vi "Get Tool Config.vi"(8 "error in (no error)":errorcluster, 10 "dummy":bool) -> (0 "error out":errorcluster, 1 "timed out?":bool, 2 "Reply Payload":T1={"Version String"="", "Tool Config"={"Tool Type"=0, "Tool SN"=0, "Tool Block"={"Encoder Size"=0, "Encoder Scale"=0, "Encoder Offset"=0, "MaxEncoder"=0, "MinEncoder"=0, "Start Delay"=0.0, "Tool Face Ref"=0.0}, "Motor Block"={"MinMotor Speed"=0, "MaxMotor Speed"=0, "Homing Speed"=90, "Jog Speed"=90, "Inspect Speed"=90, "VBlk Speed"=90, "CleaningPos"=0, "Safe Zone"=0, "Has Motor"=FALSE, "Use Home Index"=FALSE}, "Verification Block"={"Angle"=90.0, "FlankLength1"=0.0, "FlankLength2"=0.0, "Location"=0.0, "Serial Number"=0}, "Probe Block"={"nProbes"=0, "Probe Param Array"=[]}}})   [LabVIEW 2015, in "Tool Module.lvlib"]
doc: "Gets the Tool Configuration Cluster. (This copy is from the last time the app connected to the tool.)\n_____\nCreated using Delacor QMH Event Scripter 3.1.0.29."
uses:
  Tool Module.lvlib
  Get Tool Config (Reply Payload)--cluster.ctl
  Tool Config/_Configuration Cluster_v3--typedef.ctl
  Tool Config/_Tool Block Cluster_v3--typedef.ctl
  Tool Config/_Motor Block Cluster_v2--typedef.ctl
  Tool Config/_Verification Blk Cluster--typedef.ctl
  Tool Config/_ProbeConfigParams Cluster--typedef.ctl
  Tool Config/_Sensor Block Cluster--typedef.ctl
  Tool Config/_SensorConfigParams Cluster--typedef.ctl
  Get Tool Config Argument--cluster.ctl
  Tool Config/Tool Cfg.lvlib
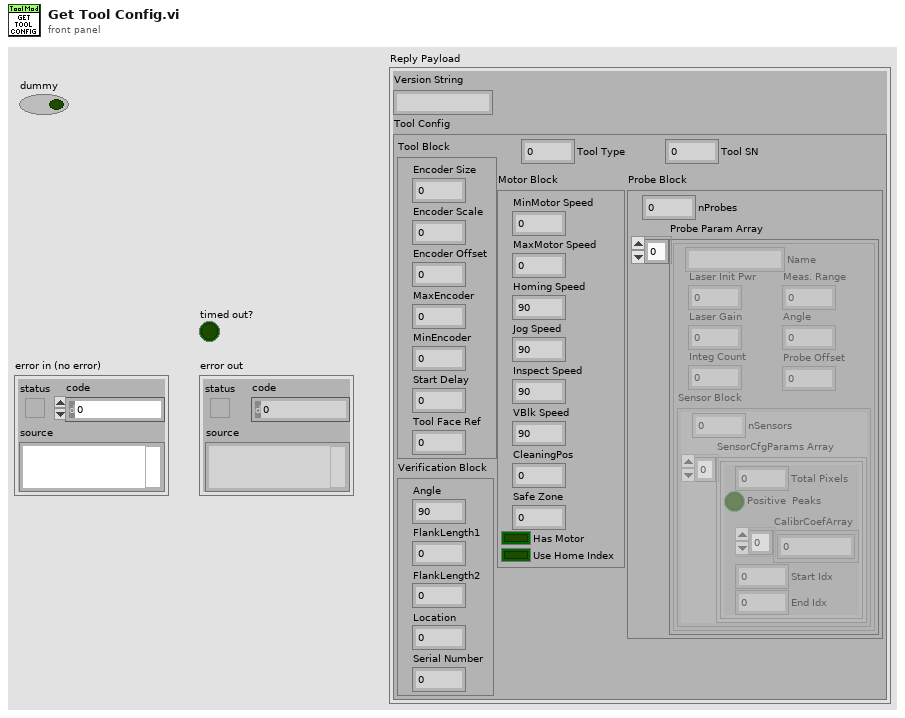
[diagram p1: front panel]
types:
  T1 = typedef "Tool Module.lvlib/Get Tool Config (Reply Payload)--cluster.ctl" = cluster{"Version String":string, "Tool Config":T2}
  T2 = typedef "Tool Cfg.lvlib/_Configuration Cluster_v3--typedef.ctl" = cluster{"Tool Type":u16, "Tool SN":u16, "Tool Block":T3, "Motor Block":T4, "Verification Block":T5, "Probe Block":cluster{"nProbes":u16, "Probe Param Array":T6[]}}
  T3 = typedef "Tool Cfg.lvlib/_Tool Block Cluster_v3--typedef.ctl" = cluster{"Encoder Size":u16, "Encoder Scale":u32, "Encoder Offset":i32, "MaxEncoder":i32, "MinEncoder":i32, "Start Delay":sgl, "Tool Face Ref":sgl}
  T4 = typedef "Tool Cfg.lvlib/_Motor Block Cluster_v2--typedef.ctl" = cluster{"MinMotor Speed":u16, "MaxMotor Speed":u16, "Homing Speed":u16, "Jog Speed":u16, "Inspect Speed":u16, "VBlk Speed":u16, "CleaningPos":i32, "Safe Zone":i32, "Has Motor":bool, "Use Home Index":bool}
  T5 = typedef "Tool Cfg.lvlib/_Verification Blk Cluster--typedef.ctl" = cluster{"Angle":sgl, "FlankLength1":sgl, "FlankLength2":sgl, "Location":sgl, "Serial Number":u16}
  T6 = typedef "Tool Cfg.lvlib/_ProbeConfigParams Cluster--typedef.ctl" = cluster{"Name":string, "Laser Init Pwr":u16, "Laser Gain":u8, "Integ Count":u16, "Meas. Range":sgl, "Angle":sgl, "Probe Offset":sgl, "Sensor Block":T7}
  T7 = typedef "Tool Cfg.lvlib/_Sensor Block Cluster--typedef.ctl" = cluster{"nSensors":u16, "SensorCfgParams Array":T8[]}
  T8 = typedef "Tool Cfg.lvlib/_SensorConfigParams Cluster--typedef.ctl" = cluster{"Total Pixels":u16, "Positive  Peaks":bool, "CalibrCoefArray":dbl[], "Start Idx":u16, "End Idx":u16}
  T9 = typedef "Tool Module.lvlib/Get Tool Config Argument--cluster.ctl" = cluster{"dummy":bool, "Wait Notifier":refnum<notifier>}
  T10 = typedef "Tool Module.lvlib/Request Events--cluster.ctl" = cluster{"Stop Module":refnum<user-event>, "Show Panel":refnum<user-event>, "Hide Panel":refnum<user-event>, "Get Module Execution Status":refnum<user-event>, "Show Diagram":refnum<user-event>, "Set OpCfg":refnum<user-event>, "Get Op Cfg":refnum<user-event>, "Test Trig 2":refnum<user-event>, "GOTO":refnum<user-event>, "Start Inspect":refnum<user-event>, "CONNECT":refnum<user-event>, "Get All Inspect Data":refnum<user-event>, "Get Inspection Limits":refnum<user-event>, "Set Inspection Limits":refnum<user-event>, "Update Status":refnum<user-event>, "Get Data Format Params":refnum<user-event>, "Start Data Monitor":refnum<user-event>, "Get FPGA Setup Params":refnum<user-event>, "Set FPGA Setup Params":refnum<user-event>, "Set Tool Config":refnum<user-event>, "Get Tool Config":refnum<user-event>, "Set Integration Count":refnum<user-event>, "Set Laser Params":refnum<user-event>, "Get Mtrl Ctrl Reg":refnum<user-event>, "Commit Ctrl Reg":refnum<user-event>, "Set Event Logger":refnum<user-event>, "Write to File":refnum<user-event>, "Read from File":refnum<user-event>, "Set Device Temp Thresholds":refnum<user-event>}
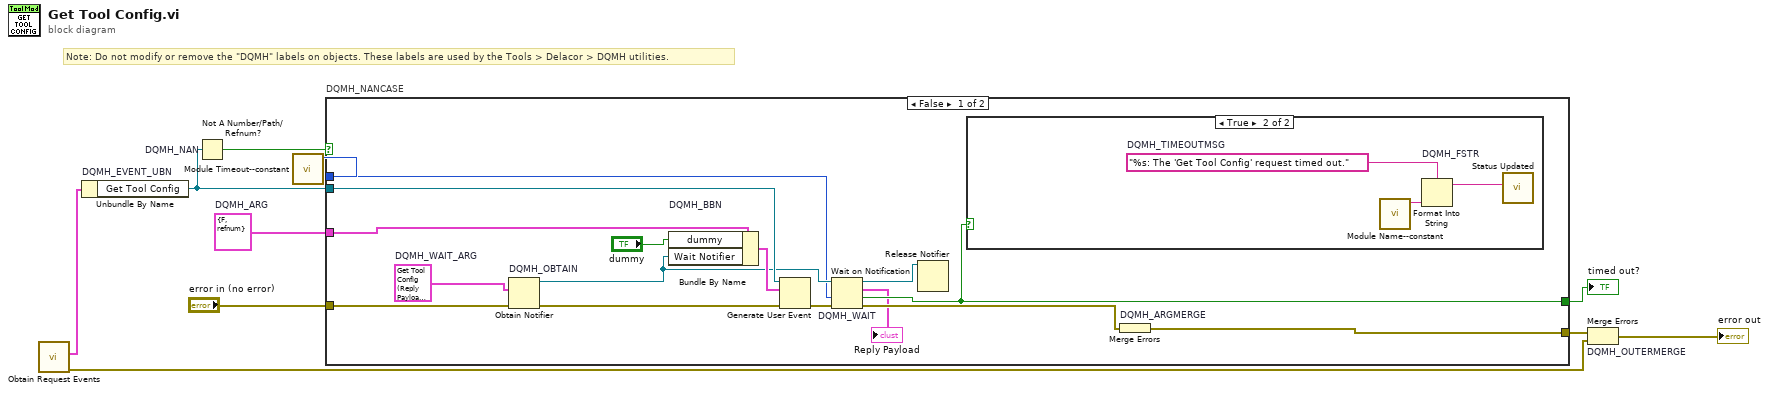
[diagram p0: block diagram]
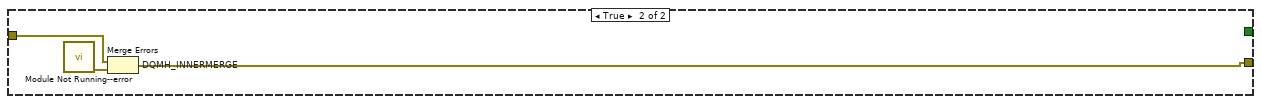
[diagram p3: hidden frame]
diagram:
  w4 = T9 {"dummy"=FALSE, "Wait Notifier"=refnum}  # DQMH_ARG
  # "Note: Do not modify or remove the \"DQMH\" labels on objects. These labels are used by the Tools > Delacor > DQMH utilities."
  n1 = call "Obtain Request Events.vi"() -> ("error out"=w2:errorcluster, "Tool Module Request Events"=w1:T10)  [unwired: 10 in]
  n2 = Unbundle By Name "DQMH_EVENT_UBN"(w1) -> ("Get Tool Config"=w8:refnum<user-event>)
  n3 = Not A Number/Path/Refnum? "DQMH_NAN"(number/path/refnum=w8) -> (NaN/Path/Refnum?=w7:bool)
  n4 = call "Module Timeout--constant.vi"() -> ("Module Timeout"=w3:i32)  [unwired: 11 in]
  n5 = case "DQMH_NANCASE" shown="False" w7 {
    tunnel: "error in (no error)" -> [w25 w31]
    tunnel: w8 -> [w23 _]
    tunnel: [w15 w30] -> w5
    tunnel: [w16 _] -> w6
    tunnel: w4 -> [w14 _]
    tunnel: w3 -> [w12 _]
    frame False {
      w20 = T1 {"Version String"="", "Tool Config"={"Tool Type"=0, "Tool SN"=0, "Tool Block"={"Encoder Size"=0, "Encoder Scale"=0, "Encoder Offset"=0, "MaxEncoder"=0, "MinEncoder"=0, "Start Delay"=0.0, "Tool Face Ref"=0.0}, "Motor Block"={"MinMotor Speed"=0, "MaxMotor Speed"=0, "Homing Speed"=90, "Jog Speed"=90, "Inspect Speed"=90, "VBlk Speed"=90, "CleaningPos"=0, "Safe Zone"=0, "Has Motor"=FALSE, "Use Home Index"=FALSE}, "Verification Block"={"Angle"=90.0, "FlankLength1"=0.0, "FlankLength2"=0.0, "Location"=0.0, "Serial Number"=0}, "Probe Block"={"nProbes"=0, "Probe Param Array"=[]}}}  # DQMH_WAIT_ARG
      n6 = Obtain Notifier "DQMH_OBTAIN"(notification data type=w20, error in (no error)=w25) -> (notifier out=w18:refnum<notifier>, error out=w21:errorcluster)  [unwired: 2 in, 1 out]
      n7 = Bundle By Name "DQMH_BBN"(cluster=w14, "dummy"="dummy", "Wait Notifier"=w18) -> (w22:T9)
      n8 = Generate User Event(user event=w23, event data cluster=w22, error in=w21) -> (error out=w24:errorcluster)  [unwired: 1 in, 1 out]
      n9 = Wait on Notification "DQMH_WAIT"(notifier=w18, timeout in ms (-1)=w12, error in (no error)=w24) -> (notifier out=w17:refnum<notifier>, notification=→"Reply Payload":T1, timed out?=w16:bool, error out=w19:errorcluster)  [unwired: 1 in]
      n10 = Release Notifier(notifier=w17) -> ()  [unwired: 2 in, 3 out]
      n11 = case shown="True" w16 {
        frame False {
        }
        frame True {
          w28 = "%s: The 'Get Tool Config' request timed out."  # DQMH_TIMEOUTMSG
          n12 = call "Module Name--constant.vi"() -> ("Module Name"=w27:string)  [unwired: 11 in]
          n13 = Format Into String "DQMH_FSTR"(format string=w28, w27) -> (resulting string=w26:string)  [unwired: 2 in, 1 out]
          n14 = call "Status Updated.vi"("Status"=w26) -> ()  [unwired: 10 in, 1 out]
        }
      }
      n15 = Merge Errors "DQMH_ARGMERGE"(w19) -> (w15:errorcluster)
    }
    frame True {
      n16 = call "Module Not Running--error.vi"() -> ("error out"=w29:errorcluster)  [unwired: 11 in]
      n17 = Merge Errors "DQMH_INNERMERGE"(w31, w29) -> (w30:errorcluster)
    }
  }
  "timed out?" <- w6
  n18 = Merge Errors "DQMH_OUTERMERGE"(w5, w2) -> (→"error out":errorcluster)
